vi "Handle Reply.vi"(7 "TcpPayload":T1, 10 "Reply Dispatch Loop Data in":T2) -> (2 "Reply Dispatch Loop Data":T2)   [LabVIEW 2020, in "Vecto.lvlib" / "TCPMessaging.lvclass"]
uses:
  TCPMessaging.lvclass
  Reply Dispatch Loop Data.ctl
  Request Registration.ctl
  lv-promises/Promises/Promise/Promise.lvclass
  lv-volatus/messages/TcpPayload/Data.ctl
  ReplyValue/ReplyValue.lvclass/ReplyValue.ctl
  ReplyValue/ReplyValue.lvclass
  TCPMessaging.lvclass/TCPMessaging.ctl
  lv-volatus/messages/TcpReply/TcpReply.lvlib
  lv-volatus/messages/TcpPayload/TcpPayload.lvlib
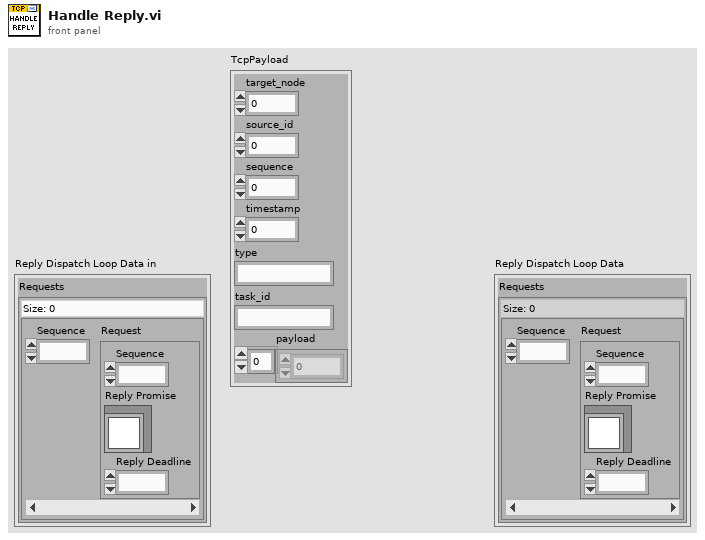
[diagram p1: front panel]
types:
  T1 = typedef "TcpPayload.lvlib/Data.ctl" = cluster{"target_node":u32, "source_id":u32, "sequence":u32, "timestamp":i64, "type":string, "task_id":string, "payload":u8[]}
  T2 = typedef "Vecto.lvlib/TCPMessaging.lvclass/Reply Dispatch Loop Data.ctl" = cluster{"Requests":map{u32, T3}}
  T3 = typedef "Vecto.lvlib/TCPMessaging.lvclass/Request Registration.ctl" = cluster{"Sequence":u32, "Reply Promise":refnum<class "Promise.lvclass">, "Reply Deadline":dbl}
  T4 = typedef "TcpReply.lvlib/Data.ctl" = cluster{"request_sequence":u32, "request_timestamp":u64, "payload":u8[], "type":string}
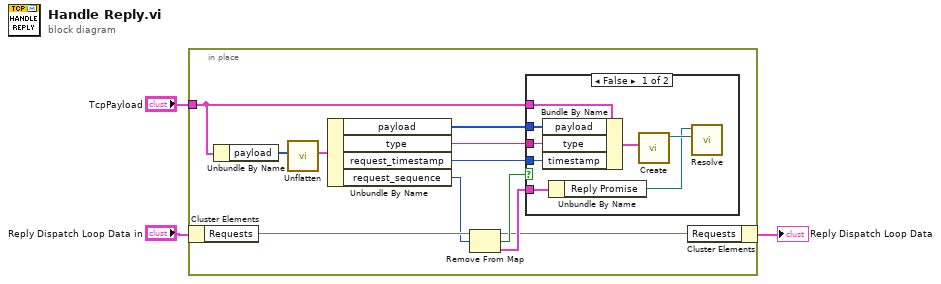
[diagram p0: block diagram]
diagram:
  n1 = in-place {
    in-place-border: "TcpPayload" -> [w5]
    n2 = in-place-cluster #1("Reply Dispatch Loop Data in") -> ("Requests"=w14:map{u32, T3})
    n3 = Unbundle By Name(w5) -> ("payload"=w13:u8[])
    n4 = call "Unflatten.vi"("Buffer"=w13) -> ("Data"=w12:T4)  [unwired: 9 in, 1 out]
    n5 = Unbundle By Name(w12) -> ("payload"=w6:u8[], "type"=w7:string, "request_timestamp"=w4:u64, "request_sequence"=w8:u32)
    n6 = Remove From Map(10:w8, 11:w14) -> (1:w10:T3, 2:w11:bool, 3:w9:map{u32, T3})
    n7 = case shown="False" w11 {
      tunnel: w10 -> [w18 _]
      tunnel: w7 -> [w20 _]
      tunnel: w6 -> [w21 _]
      tunnel: w5 -> [w22 _]
      tunnel: w4 -> [w19 _]
      frame False {
        n8 = Bundle By Name(cluster=w22, "payload"=w21, "type"=w20, "timestamp"=w19) -> (w17:T1)
        n9 = Unbundle By Name(w18) -> ("Reply Promise"=w15:refnum<class "Promise.lvclass">)
        n10 = call "Create.vi"("TcpPayload"=w17) -> ("ReplyValue out"=w16:refnum<class "ReplyValue.lvclass">)  [unwired: 10 in]
        n11 = call "Resolve.vi"("Result (None)"=w16, "Promise in"=w15) -> ()  [unwired: 8 in, 2 out]
      }
      frame True {
        # "Request is not registered. Reply could be late or bug."
      }
    }
    n12 = in-place-cluster #1("Requests"=w9) -> (→"Reply Dispatch Loop Data":T2)
  }
